vi "Day2Part2.vi"() -> ()   [LabVIEW 2024]
panel:
  out "sum":i64
  out "all rows":i64[][](array[numeric])
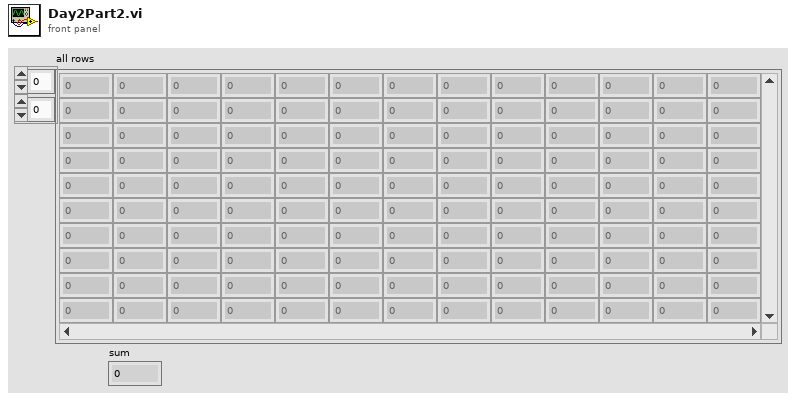
[diagram p1: front panel]
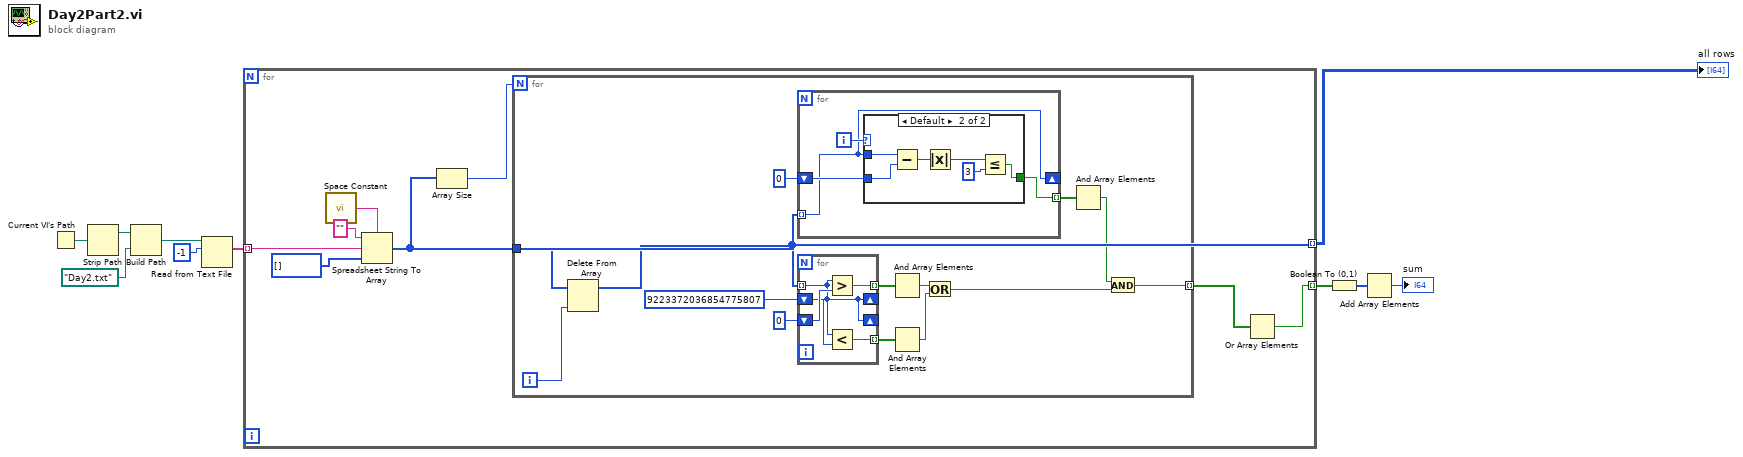
[diagram p0: block diagram]
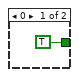
[diagram p2: hidden frame]
diagram:
  n1 = Current VI's Path() -> (path=w10:path)
  n2 = Strip Path(path=w10) -> (stripped path=w9:path)  [unwired: 1 out]
  n3 = Build Path(base path=w9, name or relative path=path "Day2.txt") -> (appended path=w4:path)
  n4 = Read from Text File(file (use dialog)=w4, count=-1) -> (text=w3:string[])  [unwired: 2 in, 3 out]
  n5 = for {
    tunnel: [w11] -> w6 mode=indexing
    tunnel: w3 -> [w18] mode=indexing
    tunnel: [w14] -> w1 mode=indexing
    n6 = call <vilib>:"Space Constant.vi"() -> ("String"=w15:string)
    n7 = Spreadsheet String To Array(delimiter (Tab)=w15, format string="", spreadsheet string=w18, array type (2D Dbl)=i64[] []) -> (array=w14:i64[])
    n8 = Array Size(array=w14) -> (size(s)=w13:i32)
    n9 = for {
      N: w13 -> [_]
      tunnel: [w26] -> w12 mode=indexing
      tunnel: w14 -> [w21]
      i -> [w20]
      n10 = Delete From Array(array=w21, index=w20) -> (array with subset deleted=w19:i64[])  [unwired: 1 in, 1 out]
      n11 = for {
        tunnel: w19 -> [w38] mode=indexing
        tunnel: [w41] -> w29 mode=indexing
        shift-right: [w38] -> _
        shift-left: i64 0 ("Numeric") -> [w40]
        i -> [w39]
        n12 = case shown="Default" w39 {
          tunnel: [TRUE w47] -> w41
          tunnel: w40 -> [_ w46]
          tunnel: w38 -> [_ w43]
          frame 0 {
          }
          frame Default {
            n13 = Subtract(x=w43, y=w46) -> (x-y=w45:i64)
            n14 = Absolute Value(x=w45) -> (abs(x)=w44:i64)
            n15 = Less Or Equal?(x=w44, y=i64 3) -> (x <= y?=w47:bool)
          }
        }
      }
      n16 = for {
        tunnel: w19 -> [w33] mode=indexing
        tunnel: [w37] -> w32 mode=indexing
        tunnel: [w36] -> w22 mode=indexing
        shift-right: [w33] -> _
        shift-left: i64 9223372036854775807 ("y") -> [w34]
        shift-right: [w33] -> _
        shift-left: i64 0 ("y") -> [w35]
        n17 = Greater?(x=w33, y=w35) -> (0:w37:bool)
        n18 = Less?(x=w33, y=w34) -> (x < y?=w36:bool)
      }
      n19 = And Array Elements(Boolean array=w32) -> (logical AND=w30:bool)
      n20 = And Array Elements(Boolean array=w22) -> (logical AND=w31:bool)
      n21 = Or(x=w30, y=w31) -> (x .or. y?=w27:bool)
      n22 = And Array Elements(Boolean array=w29) -> (logical AND=w28:bool)
      n23 = And(x=w28, y=w27) -> (x .and. y?=w26:bool)
    }
    n24 = Or Array Elements(Boolean array=w12) -> (logical OR=w11:bool)
  }
  "all rows" <- w1
  n25 = Boolean To (0,1)(Boolean=w6) -> (0, 1=w5:i16[])
  n26 = Add Array Elements(numeric array=w5) -> (sum=→"sum":i16)
